vi "Spectral Density.vi"() -> ()   [LabVIEW 2015]
uses:
  <vilib>/addons/_NISVFA/_Spectrum Processing/SVFA Spectrum Peak Search (1 Ch).vi
  <vilib>/addons/_NISVFA/_Spectrum Processing/subVIs/svfa_Spectrum Peak Search.vi
  <vilib>/addons/_NISVFA/_Shared subVIs/Common/svc_Spectrum Units.vi
  <vilib>/addons/_NISVFA/_Spectrum Processing/subVIs/svfa_Peak Rough Search Indices.vi
  <vilib>/addons/_NISVFA/_Subset FFT/SVFA Power Spectrum Subset (1 Ch).vi
  <vilib>/addons/_NISVFA/_Spectrum Processing/subVIs/svfa_Three Finger Peak Search.vi
  <vilib>/addons/_NISVFA/_Shared subVIs/Common/svc_Format Value (DBL).vi
  <vilib>/addons/_NISVFA/_Shared subVIs/Common/svc_Engineering Units to Unit Label.vi
  <vilib>/addons/_NISVFA/_Shared subVIs/Common/svc_Unit Label Lexical Class.vi
  <vilib>/addons/_NISVFA/_Shared subVIs/Common/svc_Get Weighting Enum and Labels.vi
  <vilib>/addons/_NISVFA/_Shared subVIs/Common/svc_Caller VI Returned in Error Source.vi
panel:
  out "Black Box Detected":bool
  out "Hi/Lo":dbl format="%#_13g"
  out "Hi/Lo":dbl format="%#_13g"
  out "Hi/Lo":dbl format="%#_13g"
  in  "stop 2":bool
  out "Signal 3":dbl[](array[numeric])
  out "Signal 2":dbl[](array[numeric])
  out "Signal":dbl[](array[numeric])
  out "number of peaks":i32
  in  "Peak search type":u16(ring)=1 items=["Peak Search 0", "Peak Search 1"]
  in  "PSD type":u16(ring) items=["PSD 0", "PSD 1"]
  in  "Threshold":dbl=-28.0
  in  "Min Scale":dbl
  in  "Max Scale":dbl=10000.0
  out "peaks":cluster{"freq. or order":dbl, "value":dbl}[](array[cluster])=[{"freq. or order"=99.99850804277241, "value"=-0.7926774419152083}, {"freq. or order"=1000.0, "value"=-20.789519028935615}, {"freq. or order"=2500.180930647048, "value"=-26.722435636658822}] {"value" format="%#.1g"; "freq. or order" format="%#_4g"}
  in  "stop":bool
  out "Waveform Graph":cluster{"x0":dbl, "dx":dbl, "magnitude":dbl[]}(graph)={"x0"=0.0, "dx"=10.0, "magnitude"=array[5000 elements]}
  # "Team ICARUS Acoustic Detection"
  # "Power Spectral Density"
  # "Threshold"
  # "Peaks"
  # "Magnitude"
  # "Frequency"
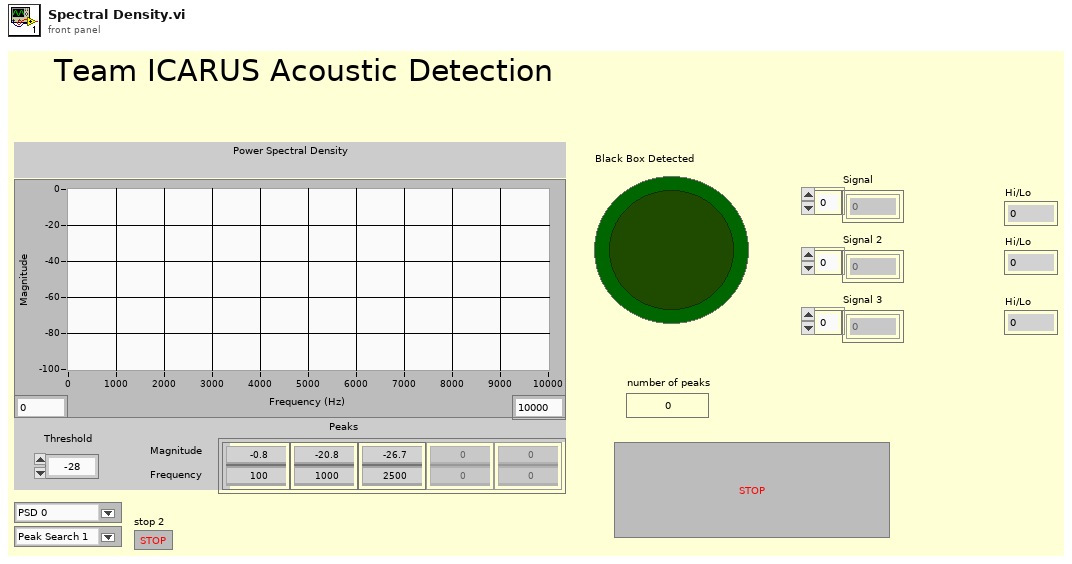
[diagram p1: front panel]
types:
  T1 = cluster{"single/multiple":enum16{"Multiple Peaks", "Single Max Peak"}, "Threshold":dbl}
  T2 = typedef "svc_Spectrum Info.ctl" = cluster{"channel name":string, "description":string, "x-axis units":T3, "spectral info":cluster{"spectrum type":T4, "linear/dB":enum16{"linear", "dB"}, "window":u16, "window size":i32, "FFT size":i32}, "engineering units":T5, "custom label":string, "dB reference [EU]":dbl, "peak units":enum16{"rms", "peak", "peak-peak"}, "weighting filter":T6, "spectral density?":bool, "unit label":string, "spectrum skewed?":bool, "complimentary spectrum units":T7}
  T3 = typedef "svc_X-Axis Units.ctl" = u16
  T4 = typedef "svc_Spectrum Type.ctl" = enum16{"FFT Spectrum [complex]", "Amplitude [Magnitude]", "Power [Magnitude^2]", "Cross Spectrum [complex]", "Frequency Response [Complex]"}
  T5 = typedef "svc_Engineering Units Text Ring.ctl" = u16
  T6 = typedef "svc_Weighting Filter Text Ring.ctl" = u16
  T7 = typedef "svc_Complimentary Spectrum Units.ctl" = enum16{"none", "radians", "degrees", "cycles", "imaginary"}
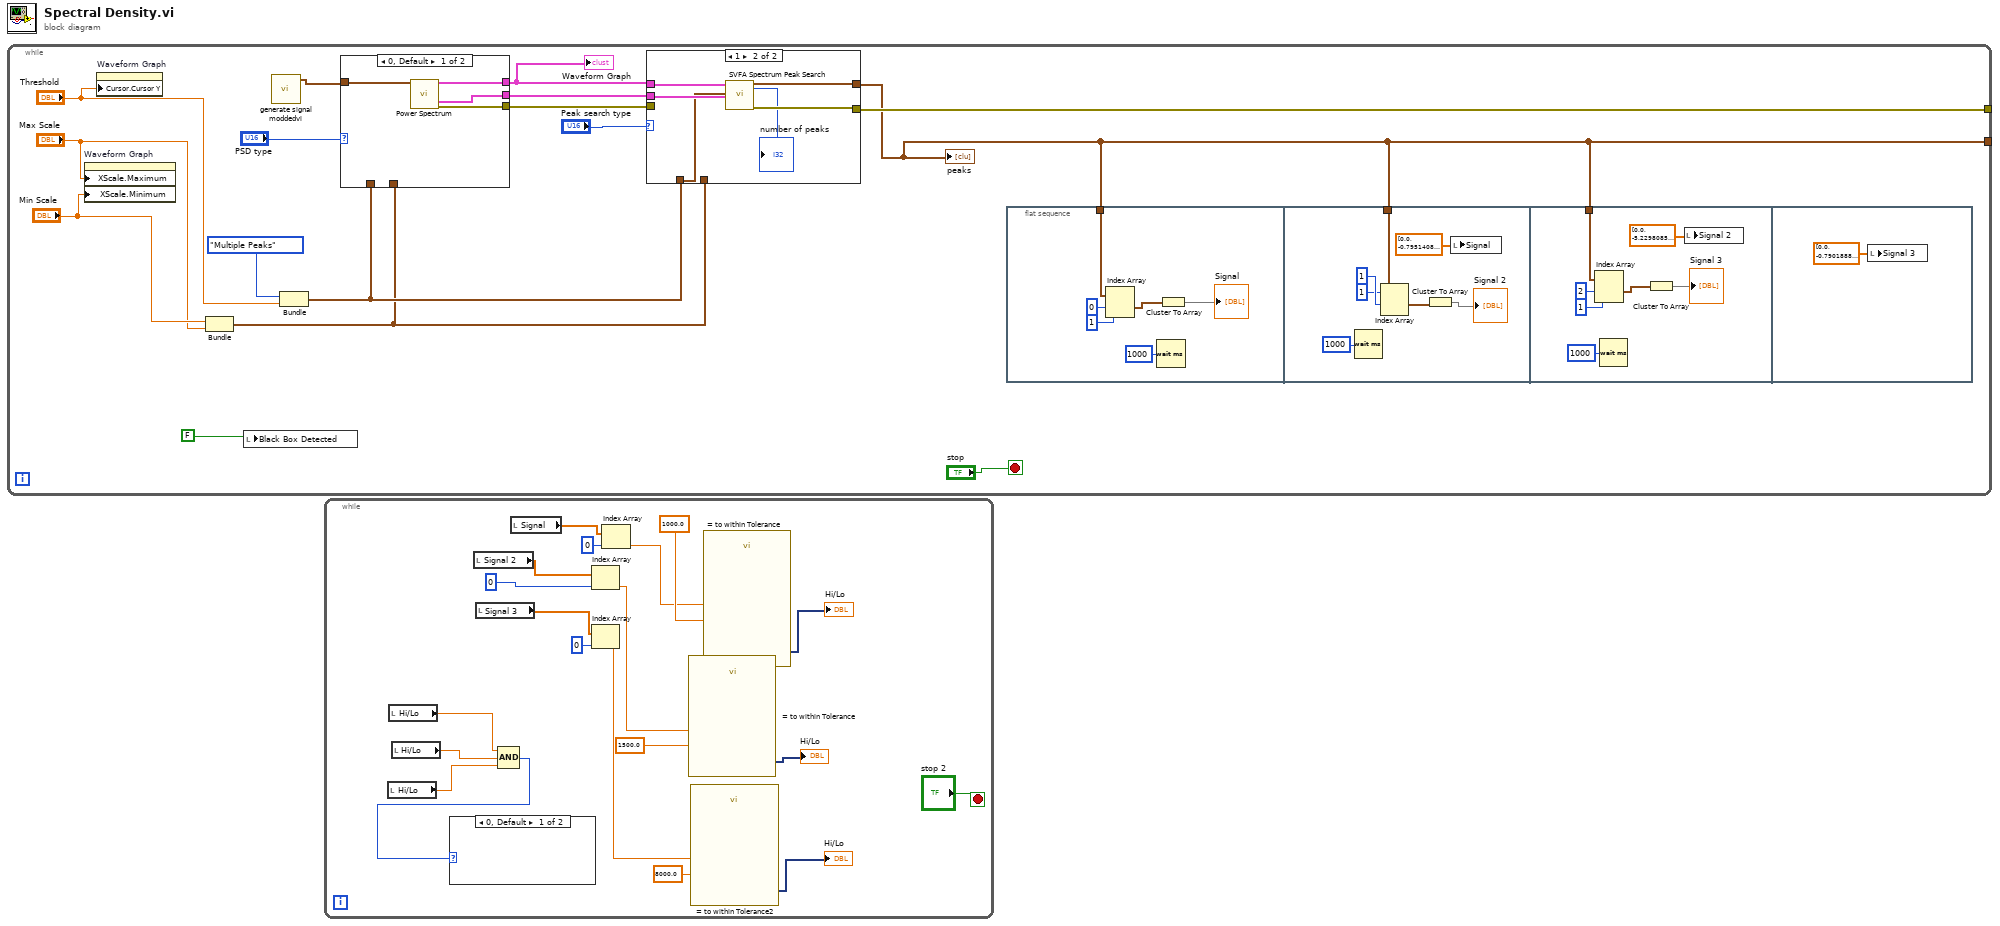
[diagram p0: block diagram]
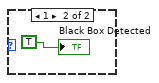
[diagram p2: hidden frame]
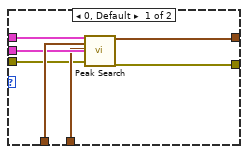
[diagram p3: hidden frame]
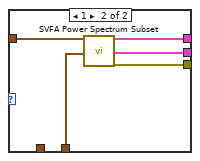
[diagram p4: hidden frame]
diagram:
  n1 = while {
    tunnel: [w5] -> _
    tunnel: [w1] -> _
    stop <- "stop" stop-if-true
    n2 = property on="Waveform Graph" class="WFGraph (strict)"("XScale.Maximum"="Max Scale", "XScale.Minimum"="Min Scale") -> ()  [unwired: 2 in, 2 out]
    n3 = property on="Waveform Graph" class="WFGraph (strict)"("Cursor.Cursor Y"="Threshold") -> ()  [unwired: 2 in, 2 out]
    n4 = Bundle("Min Scale"="Min Scale", "Max Scale"="Max Scale") -> (w9:cluster{"Min Scale":dbl, "Max Scale":dbl})  [unwired: 1 in]
    n5 = local write "Black Box Detected"(FALSE) -> ()
    n6 = call "generate signal moddedvi.vi"() -> ("Waveform Graph 5"=w4:waveform(dbl))  [unwired: 11 in]
    n7 = Bundle("single/multiple"=enum16{"Multiple Peaks", "Single Max Peak"}."Multiple Peaks", "Threshold"="Threshold") -> (w10:T1)  [unwired: 1 in]
    n8 = case shown="0, Default" "PSD type" {
      tunnel: w4 -> [w54 w57]
      tunnel: [w53 w59] -> w13
      tunnel: [w52 w58] -> w14
      tunnel: w10 -> [_ _]
      tunnel: w9 -> [_ w56]
      tunnel: [w51 w55] -> w6
      frame 0, Default {
        n9 = call "Power Spectrum"("input signal"=w54) -> ("spectrum"=w53:cluster{"x0":dbl, "dx":dbl, "magnitude":dbl[]}, "spectrum info"=w52:T2, "error out"=w51:errorcluster)  [unwired: 13 in, 3 out]
      }
      frame 1 {
        n10 = call-poly <vilib>:"SVFA Power Spectrum Subset.vi"("scaled signal [EU]"=w57, "frequency range"=w56) -> ("power spectrum [dB EU]"=w59:cluster{"f0":dbl, "df":dbl, "magnitude":dbl[]}, "spectrum info"=w58:T2, "error out"=w55:errorcluster)  [unwired: 12 in, 3 out]
      }
    }
    "Waveform Graph" <- w13
    n11 = case shown="1" "Peak search type" {
      tunnel: w13 -> [w44 w50]
      tunnel: w10 -> [w43 w47]
      tunnel: w14 -> [w42 w49]
      tunnel: w9 -> [w41 _]
      tunnel: [w40 w48] -> w1
      tunnel: w6 -> [w39 _]
      tunnel: [w38 w46] -> w5
      frame 0, Default {
        n12 = call "Peak Search"("input spectrum"=w44, "peak search settings"=w43, "frequency range"=w41, "spectrum info"=w42, "error in"=w39) -> ("peaks"=w40:cluster{"freq. or order":dbl, "value":dbl}[], "error out"=w38:errorcluster)  [unwired: 11 in, 2 out]
      }
      frame 1 {
        n13 = call-poly <vilib>:"SVFA Spectrum Peak Search.vi"("spectrum"=w50, "peak search settings"=w47, "spectrum info in"=w49) -> ("peaks"=w48:cluster{"freq. or order":dbl, "value":dbl}[], "number of peaks"=→"number of peaks":i32, "error out"=w46:errorcluster)  [unwired: 12 in, 2 out]
      }
    }
    "peaks" <- w1
    n14 = flat-sequence {
      tunnel: w1 -> [w20]
      tunnel: w1 -> [w26]
      tunnel: w1 -> [w33]
      frame #0 {
        n15 = Index Array(array=w20, index #1=0 ("index"), index #2=1 ("index")) -> (element #1=w19:cluster{"freq. or order":dbl, "value":dbl})  [unwired: 1 out]
        n16 = Wait (ms)(milliseconds to wait=u32 1000) -> ()  [unwired: 1 out]
        n17 = Cluster To Array(cluster=w19) -> (array=→"Signal":dbl[])
      }
      frame #1 {
        n18 = Wait (ms)(milliseconds to wait=u32 1000) -> ()  [unwired: 1 out]
        n19 = Index Array(array=w26, index #1=1 ("index"), index #2=1 ("index")) -> (element #1=w25:cluster{"freq. or order":dbl, "value":dbl})  [unwired: 1 out]
        n20 = Cluster To Array(cluster=w25) -> (array=→"Signal 2":dbl[])
        n21 = local write "Signal"(dbl[] [0.0, -0.795140880009273] ("Signal")) -> ()
      }
      frame #2 {
        n22 = Index Array(array=w33, index #1=2 ("index"), index #2=1 ("index")) -> (element #1=w32:cluster{"freq. or order":dbl, "value":dbl})  [unwired: 1 out]
        n23 = Wait (ms)(milliseconds to wait=u32 1000) -> ()  [unwired: 1 out]
        n24 = Cluster To Array(cluster=w32) -> (array=→"Signal 3":dbl[])
        n25 = local write "Signal 2"(dbl[] [0.0, -5.229808512543559] ("Signal 2")) -> ()
      }
      frame #3 {
        n26 = local write "Signal 3"(dbl[] [0.0, -0.7901888756141631] ("Signal 3")) -> ()
      }
    }
  }
  n27 = while {
    stop <- "stop 2" stop-if-true
    n28 = local read "Hi/Lo"() -> (w61:dbl)
    n29 = local read "Hi/Lo"() -> (w63:dbl)
    n30 = local read "Hi/Lo"() -> (w62:dbl)
    n31 = local read "Signal 2"() -> (w76:dbl[])
    n32 = local read "Signal 3"() -> (w75:dbl[])
    n33 = Compound Arithmetic op=AND(w63, w62, w61) -> (w60:i32)
    n34 = case shown="0, Default" w60 {
      frame 0, Default {
      }
      frame 1 {
        "Black Box Detected" <- TRUE
      }
    }
    n35 = local read "Signal"() -> (w78:dbl[])
    n36 = Index Array(array=w76, index=0) -> (element=w69:dbl)
    n37 = Index Array(array=w75, index=0) -> (element=w68:dbl)
    n38 = Index Array(array=w78, index=0) -> (element=w70:dbl)
    n39 = call "= to within Tolerance"("Constant Value to Compare Against"=1500.0, "Operand 1"=w69) -> ("Result"=→"Hi/Lo":dynamicdata)  [unwired: 8 in, 1 out]
    n40 = call "= to within Tolerance2"("Constant Value to Compare Against"=8000.0, "Operand 1"=w68) -> ("Result"=→"Hi/Lo":dynamicdata)  [unwired: 8 in, 1 out]
    n41 = call "= to within Tolerance"("Constant Value to Compare Against"=1000.0, "Operand 1"=w70) -> ("Result"=→"Hi/Lo":dynamicdata)  [unwired: 8 in, 1 out]
  }
